vi "Global Var.vi"() -> ()   [LabVIEW 2013]
panel:
  in  "Z Desplazamiento Unidad":i32
  in  "Y Desplazamiento Unidad":i32
  in  "X Desplazamiento Unidad":i32
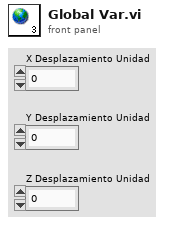
[diagram p1: front panel]
diagram:
